vi "Analytical Inverse Kinematics.vi"   [LabVIEW 2017, in "NI_Robotics_AnalyticKinematics.lvlib"]
doc: "Returns the joint angles of a 6R, 5R, or SCARA arm given the posture of the end effector relative to the arm base. Wire data to the <B>X</B><B>_serial arm in</B> input, where <B>X</B> is the arm type, to determine the polymorphic instance to use or manually select the instance."
uses:
  <vilib>/robotics/Kinematics/Analytical/NI_Robotics_AnalyticKinematics.lvlib
  <vilib>/robotics/Kinematics/Analytical/6R/Type 1/NI_Robotics_6R Type 1 Serial Arm Class.lvclass
  <vilib>/robotics/Kinematics/Analytical/SCARA/NI_Robotics_SCARA Serial Arm Class.lvclass
  <vilib>/robotics/Kinematics/Analytical/6R/Type 2/NI_Robotics_6R Type 2 Serial Arm Class.lvclass
  <vilib>/robotics/Kinematics/Analytical/6R/Type 3/NI_Robotics_6R Type 3 Serial Arm Class.lvclass
  <vilib>/robotics/Kinematics/Analytical/5R/Type 1/NI_Robotics_5R Type 1 Serial Arm Class.lvclass
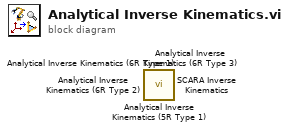
[diagram p0: block diagram]
diagram:
  n1 = call <vilib>:"Analytical Inverse Kinematics (5R Type 1).vi"() -> ()  [unwired: 8 in, 4 out]
  n2 = call <vilib>:"Analytical Inverse Kinematics (6R Type 3).vi"() -> ()  [unwired: 8 in, 4 out]
  n3 = call <vilib>:"Analytical Inverse Kinematics (6R Type 2).vi"() -> ()  [unwired: 8 in, 4 out]
  n4 = call <vilib>:"SCARA Inverse Kinematics.vi"() -> ()  [unwired: 9 in, 3 out]
  n5 = call <vilib>:"Analytical Inverse Kinematics (6R Type 1).vi"() -> ()  [unwired: 8 in, 4 out]
